vi "Load Program From File.vi"(8 "Error In":errorcluster, 10 "Program Path":path, 11 "Device In":T2) -> (0 "Error Out":errorcluster, 2 "Program Handle":T1, 3 "Device Out":T2)   [LabVIEW 2012]
doc: "Loads a specified program from disk. If the path is not valid or empty, a GUI is launched to help configure a program.\n\nThe GUI has options to load a program, save a program, compile a program, cancel the GUI, or finish the program. Please see the manual for more details."
uses:
  Non-User VIs/Controls/Device ID.ctl
  Non-User VIs/Controls/Program Handle.ctl
  OpenCLV x64.lvlib
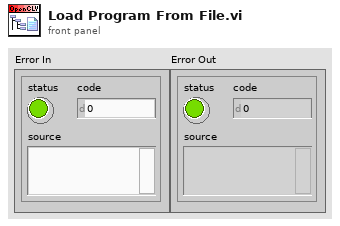
[diagram p1: front panel]
types:
  T1 = typedef "OpenCLV x64.lvlib/Program Handle.ctl" = u64
  T2 = typedef "OpenCLV x64.lvlib/Device ID.ctl" = u64
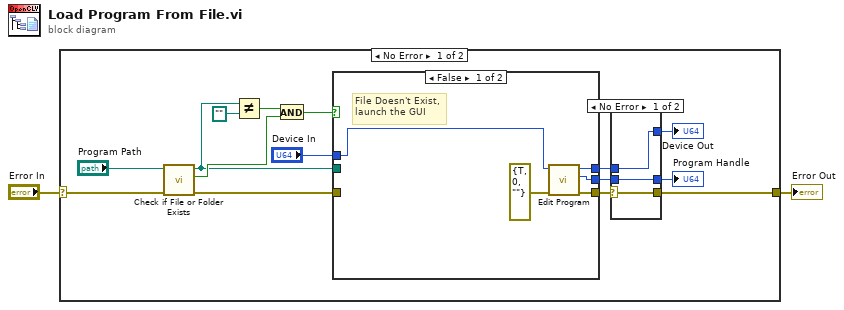
[diagram p0: block diagram]
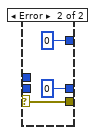
[diagram p2: hidden frame]
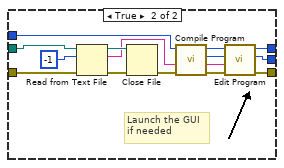
[diagram p3: hidden frame]
diagram:
  n1 = case shown="No Error" "Error In" {
    selector: "Error In" -> [w14 w44]
    tunnel: [w5 w44] -> w1
    frame No Error {
      n2 = call <vilib>:"Check if File or Folder Exists.vi"("error in (no error)"=w14, "path"="Program Path") -> ("error out"=w15:errorcluster, "file or folder exists?"=w11:bool, "dup path"=w9:path)  [unwired: 7 in]
      n3 = Not Equal?(x=w9, y=path "") -> (x != y?=w12:bool)
      n4 = And(x=w12, y=w11) -> (x .and. y?=w13:bool)
      n5 = case shown="False" w13 {
        tunnel: [w28 w36] -> w8
        tunnel: "Device In" -> [w27 w43]
        tunnel: w9 -> [_ w42]
        tunnel: w15 -> [_ w41]
        tunnel: [w25 w35] -> w7
        tunnel: [w26 w34] -> w6
        frame False {
          # "File Doesn't Exist,\nlaunch the GUI"
          n6 = call "Edit Program.vi"("Error In"=errorcluster {"status"=TRUE, "code"=0, "source"=""}, "Device In"=w27) -> ("Error Out"=w28:errorcluster, "Program Handle"=w25:T1, "Device Out"=w26:T2)  [unwired: 7 in]
        }
        frame True {
          # "Launch the GUI\nif needed"
          n7 = Read from Text File(file (use dialog)=w42, count=-1, error in=w41) -> (refnum out=w33:refnum<file>, text=w30:string, error out=w32:errorcluster)  [unwired: 1 in, 1 out]
          n8 = Close File(refnum=w33, error in=w32) -> (error out=w31:errorcluster)  [unwired: 1 out]
          n9 = call "Compile Program.vi"("error in (no error)"=w31, "OpenCL Source Code"=w30, "Device In in"=w43) -> ("error out"=w39:errorcluster, "OpenCL Source Code Out"=w29:string, "Program Handle"=w37:T1, "Device Out"=w38:T2)  [unwired: 5 in]
          n10 = call "Edit Program.vi"("Error In"=w39, "Program Source"=w29, "Program Handle"=w37, "Device In"=w38) -> ("Error Out"=w36:errorcluster, "Program Handle"=w35:T1, "Device Out"=w34:T2)  [unwired: 5 in]
        }
      }
      n11 = case shown="No Error" w8 {
        selector: w8 -> [w20 w23]
        tunnel: w6 -> [w19 _]
        tunnel: w7 -> [w18 _]
        tunnel: [w20 w23] -> w5
        tunnel: [w19 T2 0 ("Device Out")] -> w4
        tunnel: [w18 T1 0 ("Program Handle")] -> w3
        frame No Error {
        }
        frame Error {
        }
      }
      "Program Handle" <- w3
      "Device Out" <- w4
    }
    frame Error {
    }
  }
  "Error Out" <- w1
